vi "Pre-Smite Hook.vi"(8 "Error In":errorcluster) -> (0 "Error Out":errorcluster)   [LabVIEW 2018, in "Tests.lvlib" / "Toolkit.lvlib" / "Integration.lvlib"]
uses:
  Integration.lvlib
  Support/Smite Target.vi
  Hooks/Pre-Smite.vi
  <vilib>/addons/_JKI Toolkits/Caraya/classes/Test/Test.lvclass
  Tests.lvlib
  <vilib>/addons/_JKI Toolkits/Caraya/classes/Assert/Assert.lvclass
  src/Toolkit/Toolkit.lvlib
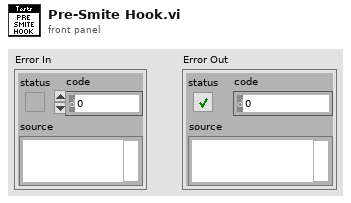
[diagram p1: front panel]
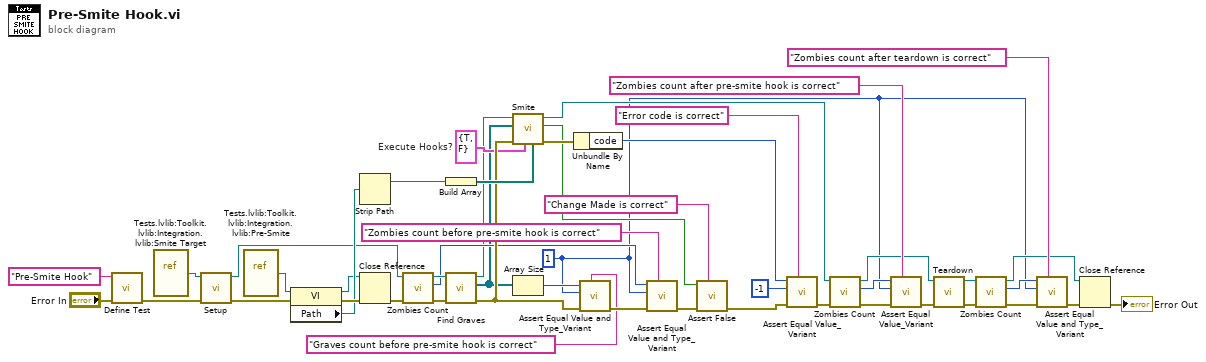
[diagram p0: block diagram]
diagram:
  w1 = 1 ("size(s)")
  w18 = cluster{"Pre":bool, "Post":bool} {"Pre"=TRUE, "Post"=FALSE}  # Execute Hooks?
  n1 = call <vilib>:"Define Test.vi"("error in (no error)"="Error In", "Label (VI Title)"="Pre-Smite Hook") -> ("error out"=w43:errorcluster)  [unwired: 9 in]
  n2 = vi-ref "Tests.lvlib:Toolkit.lvlib:Integration.lvlib:Smite Target.vi"() -> (w7:refnum<vi>)
  n3 = call "Setup.vi"("Error In"=w43, "VI In"=w7) -> ("Error Out"=w35:errorcluster, "VI Out"=w27:refnum<vi>)  [unwired: 8 in]
  n4 = vi-ref "Tests.lvlib:Toolkit.lvlib:Integration.lvlib:Pre-Smite.vi"() -> (w2:refnum<vi>)
  n5 = property class="VI"(reference=w2, error in=w35) -> (reference out=w31:refnum<vi>, error out=w34:errorcluster, "Path"=w33:path)
  n6 = Strip Path(path=w33) -> (stripped path=w32:path)  [unwired: 1 out]
  n7 = Close Reference(reference=w31, error in (no error)=w34) -> (error out=w14:errorcluster)
  n8 = call "Zombies Count.vi"("Error In"=w14, "Test Target In"=w27) -> ("Error Out"=w13:errorcluster, "Zombies Count"=w8:i32, "Test Target Out"=w15:refnum<vi>)  [unwired: 7 in]
  n9 = Build Array(w32) -> (w28:path[])
  n10 = call "Find Graves.vi"("Error In"=w13, "VI In"=w15) -> ("Error Out"=w26:errorcluster, "Graves"=w5:refnum<vi>[], "VI Out"=w6:refnum<vi>)  [unwired: 7 in]
  n11 = call "Smite.vi"("Hook Search Path"=w28, "Execute Hooks?"=w18, "Error In"=w26, "Graves"=w5, "VI In"=w6) -> ("Error Out"=w24:errorcluster, "Change Made?"=w3:bool, "VI Out"=w4:refnum<vi>)  [unwired: 4 in]
  n12 = Array Size(array=w5) -> (size(s)=w25:i32)
  n13 = Unbundle By Name(w24) -> ("code"=w30:i32)
  n14 = call <vilib>:"Assert Equal Value and Type_Variant.vi"("Label"="Graves count before pre-smite hook is correct", "error in (no error)"=w26, "Y"=w1, "X"=w25) -> ("error out"=w12:errorcluster)  [unwired: 7 in]
  n15 = call <vilib>:"Assert Equal Value and Type_Variant.vi"("Label"="Zombies count before pre-smite hook is correct", "error in (no error)"=w12, "Y"=w1, "X"=w8) -> ("error out"=w11:errorcluster)  [unwired: 7 in]
  n16 = call <vilib>:"Assert False.vi"("Label"="Change Made is correct", "error in (no error)"=w11, "False?"=w3) -> ("error out"=w17:errorcluster)  [unwired: 8 in]
  n17 = call <vilib>:"Assert Equal Value_Variant.vi"("Label"="Error code is correct", "error in (no error)"=w17, "Y"=-1 ("code"), "X"=w30) -> ("error out"=w23:errorcluster)  [unwired: 7 in]
  n18 = call "Zombies Count.vi"("Error In"=w23, "Test Target In"=w4) -> ("Error Out"=w22:errorcluster, "Zombies Count"=w21:i32, "Test Target Out"=w20:refnum<vi>)  [unwired: 7 in]
  n19 = call <vilib>:"Assert Equal Value_Variant.vi"("Label"="Zombies count after pre-smite hook is correct", "error in (no error)"=w22, "Y"=w1, "X"=w21) -> ("error out"=w19:errorcluster)  [unwired: 7 in]
  n20 = call "Teardown.vi"("Error In"=w19, "VI In"=w20) -> ("Error Out"=w38:errorcluster, "VI Out"=w40:refnum<vi>)  [unwired: 8 in]
  n21 = call "Zombies Count.vi"("Error In"=w38, "Test Target In"=w40) -> ("Error Out"=w37:errorcluster, "Zombies Count"=w36:i32, "Test Target Out"=w39:refnum<vi>)  [unwired: 7 in]
  n22 = call <vilib>:"Assert Equal Value and Type_Variant.vi"("Label"="Zombies count after teardown is correct", "error in (no error)"=w37, "Y"=w1, "X"=w36) -> ("error out"=w42:errorcluster)  [unwired: 7 in]
  n23 = Close Reference(reference=w39, error in (no error)=w42) -> (error out=→"Error Out":errorcluster)
